vi "GHV232 CRAB Query PS.vi"(8 "error in (no error)":errorcluster, 9 "Version":bool, 11 "VISA resource name":refnum<visa-resource-name>) -> (0 "error out":errorcluster, 3 "VISA resource name 2":refnum<visa-resource-name>)   [LabVIEW 2017]
panel:
  # "This VI sends a query command unless\nthe firmware verion button is true."
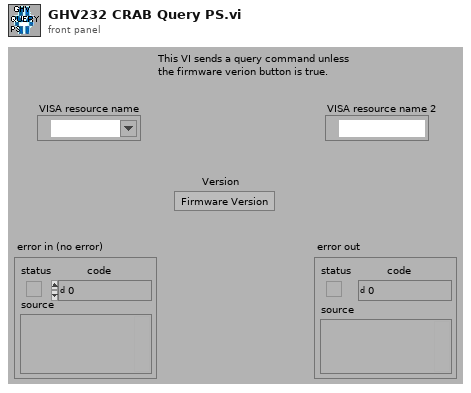
[diagram p1: front panel]
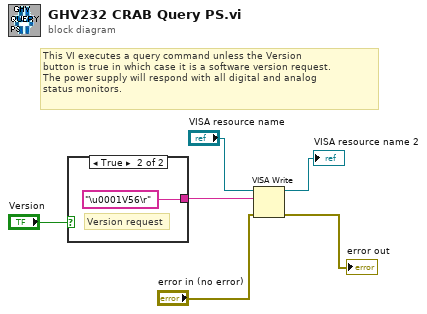
[diagram p0: block diagram]
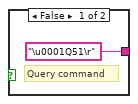
[diagram p2: hidden frame]
diagram:
  # "This VI executes a query command unless the Version\nbutton is true in which case it is a software version request.\nThe power supply will respond with all digital and analog \nstatus monitors."
  n1 = case shown="True" "Version" {
    tunnel: ["\u0001Q51\r" "\u0001V56\r"] -> w6
    frame False {
      # "Query command"
    }
    frame True {
      # "Version request"
    }
  }
  n2 = VISA Write(VISA resource name="VISA resource name", write buffer=w6, error in (no error)="error in (no error)") -> (VISA resource name out=→"VISA resource name 2":refnum<visa-resource-name>, error out=→"error out":errorcluster)  [unwired: 1 out]
